vi "Synth Program.vi"(8 "Error In":errorcluster, 10 "Init":bool=TRUE, 11 "User configuration":T3={"DAQmx Device"="", "Variable amplitude frequency"=0.0, "Fixed amplitude frequency"=0.0, "Amplitude"=0.0, "Clock multiplier"=0, "Channel names (variable F)"=[], "Channel names (fixed F)"=[], "Group"="p", "Auto-update other modules"=FALSE, "Recorder module"="", "Lock-in module "=""} {"Amplitude" format="%#_6pV"; "Fixed amplitude frequency" format="%#_6pHz"; "Variable amplitude frequency" format="%#_6pHz"}) -> (0 "Error Out":errorcluster, 1 "Lockin parameters array":T1[](array[typedef]) {"DDS clock" format="%_17pHz"; "DDS modulus" format="0x%x (%d)"; "Phase" format="%#_gdeg"; "Frequency" format="%_17pHz"}, 2 "Actual ratios":T2 {"Clock" format="%_20p"; "F2" format="%_20p"; "F1" format="%_20p"; "Clock/F2" format="%_20g"; "Clock/F1" format="%_20g"}, 3 "Actual clock":ext format="%_20p")   [LabVIEW 2016]
uses:
  NHMFL Synthesizer Configuration.ctl
  Actual Settings.ctl
  SoftwareLockin/Lockin Parameters.ctl
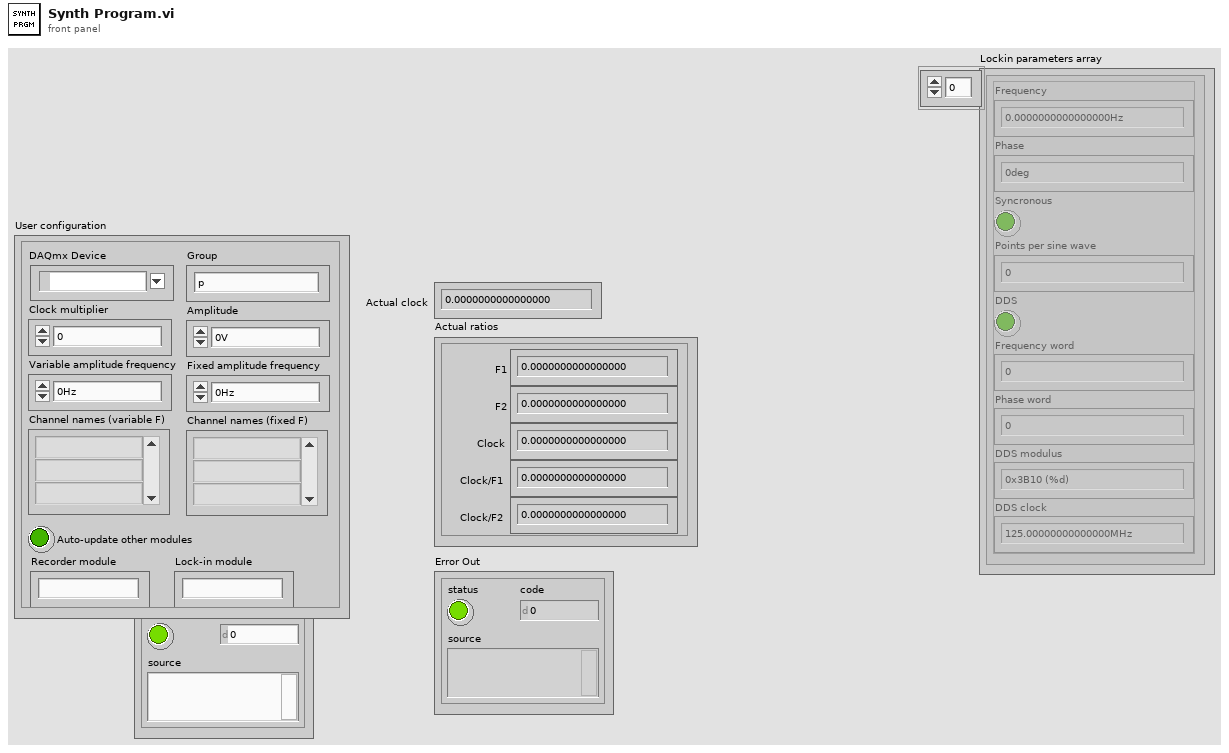
[diagram p1: front panel]
types:
  T1 = typedef "Lockin Parameters.ctl" = cluster{"Frequency":dbl, "Phase":dbl, "Syncronous":bool, "Points per sine wave":i32, "DDS":bool, "Frequency word":u32, "Phase word":u32, "DDS modulus":i64, "DDS clock":dbl}
  T2 = typedef "Actual settings.ctl" = cluster{"Clock/F1":ext, "Clock/F2":ext, "F1":ext, "F2":ext, "Clock":ext}
  T3 = typedef "NHMFL Synthesizer Configuration.ctl" = cluster{"DAQmx Device":tag, "Variable amplitude frequency":dbl, "Fixed amplitude frequency":dbl, "Amplitude":dbl, "Clock multiplier":i32, "Channel names (variable F)":string[], "Channel names (fixed F)":string[], "Group":string, "Auto-update other modules":bool, "Recorder module":string, "Lock-in module ":string}
  T4 = enum16{"Direct, clock*f1", "Direct, clock*f2", "Heterodyne"}
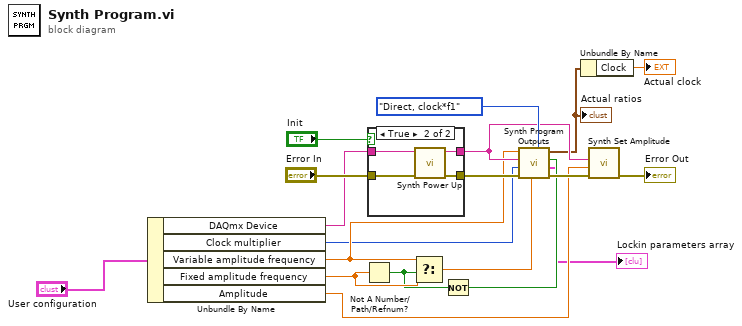
[diagram p0: block diagram]
diagram:
  n1 = Unbundle By Name("User configuration") -> ("DAQmx Device"=w3:tag, "Clock multiplier"=w2:i32, "Variable amplitude frequency"=w8:dbl, "Fixed amplitude frequency"=w6:dbl, "Amplitude"=w12:dbl)
  n2 = Not A Number/Path/Refnum?(number/path/refnum=w6) -> (NaN/Path/Refnum?=w5:bool)
  n3 = case shown="True" "Init" {
    tunnel: w3 -> [w21 w25]
    tunnel: "Error In" -> [w20 w24]
    tunnel: [w21 w23] -> w14
    tunnel: [w20 w22] -> w17
    frame False {
    }
    frame True {
      n4 = call "Synth Power Up.vi"("Error In"=w24, "DAQmx Device Name"=w25) -> ("Error Out"=w22:errorcluster, "DAQmx Device Name out"=w23:tag)  [unwired: 8 in]
    }
  }
  n5 = Select(t=w8, s=w5, f=w6) -> (s? t:f=w7:dbl)
  n6 = Not(x=w5) -> (.not. x?=w4:bool)
  n7 = call "Synth Program Outputs.vi"("Match clocks"=w4, "Mode"=T4."Direct, clock*f1", "IF (Hz)"=w7, "error in (no error)"=w17, "Clock Multiplier"=w2, "DAQmx Device Name"=w14, "f (Hz)"=w8) -> ("error out"=w13:errorcluster, "Lockin parameters array"=→"Lockin parameters array":T1[], "Actual ratios"=w11:T2)  [unwired: 2 in]
  "Actual ratios" <- w11
  n8 = Unbundle By Name(w11) -> ("Clock"=→"Actual clock":ext)
  n9 = call "Synth Set Amplitude.vi"("error in (no error)"=w13, "0 to 2.1 VRMS"=w12, "DAQmx Device Name"=w14) -> ("error out"=→"Error Out":errorcluster)  [unwired: 8 in]
